vi "drawHorizontalRange.vi"(8 "Y 2":i32, 9 "Y":i32, 10 "Xmax":i32, 11 "picture":picture) -> (3 "new picture":picture)   [LabVIEW 2016]
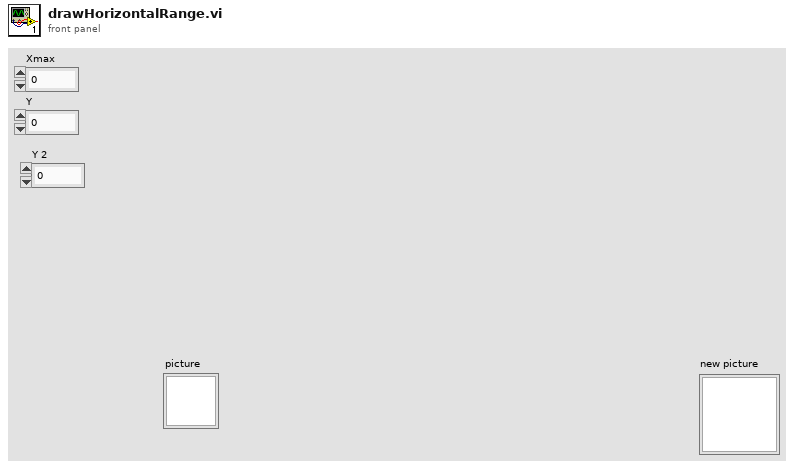
[diagram p1: front panel]
types:
  T1 = cluster{"Width":u16, "Style":enum32{"Solid", "Dash", "Dot", "DashDot", "DashDotDot"}}
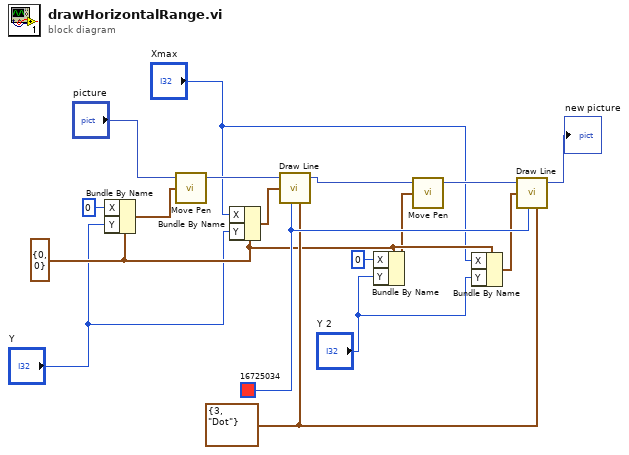
[diagram p0: block diagram]
diagram:
  w10 = cluster{"X":i32, "Y":i32} {"X"=0, "Y"=0} ("Mouse Position")
  w13 = T1 {"Width"=3, "Style"=enum."Dot"} ("pen")
  w14 = u32 16725034 ("color(black)")
  n1 = Bundle By Name(cluster=w10, "X"=0, "Y"="Y") -> (w4:cluster{"X":i32, "Y":i32})
  n2 = call <vilib>:"Move Pen.vi"("new position"=w4, "picture"="picture") -> ("new picture"=w17:picture)  [unwired: 3 in]
  n3 = Bundle By Name(cluster=w10, "X"="Xmax", "Y"="Y") -> (w3:cluster{"X":i32, "Y":i32})
  n4 = call <vilib>:"Draw Line.vi"("picture"=w17, "end point"=w3, "color(black)"=w14, "pen"=w13) -> ("new picture"=w15:picture)  [unwired: 5 in]
  n5 = Bundle By Name(cluster=w10, "X"=0, "Y"="Y 2") -> (w2:cluster{"X":i32, "Y":i32})
  n6 = call <vilib>:"Move Pen.vi"("new position"=w2, "picture"=w15) -> ("new picture"=w16:picture)  [unwired: 3 in]
  n7 = Bundle By Name(cluster=w10, "X"="Xmax", "Y"="Y 2") -> (w1:cluster{"X":i32, "Y":i32})
  n8 = call <vilib>:"Draw Line.vi"("picture"=w16, "end point"=w1, "color(black)"=w14, "pen"=w13) -> ("new picture"=→"new picture":picture)  [unwired: 5 in]
